vi "Garland_SB parse navigation string.vi"(6 "Header":string="T", 8 "Nav String":string="$,G,43,13,230,P,10,20,120,T,10,10,330,L,14,36,110,A,3,5,B,7,8,C,16,20,D,-1,-1,S,08,12,234\r") -> (0 "Valid?":bool, 1 "angle":i32, 2 "y":i32, 3 "x":i32)   [LabVIEW 2013]
doc: "This VI will parse the Tug navigation string for the Tug letters, A for example, and the time, T. It returns a cluster with the Tug / Time and three values as decimals."
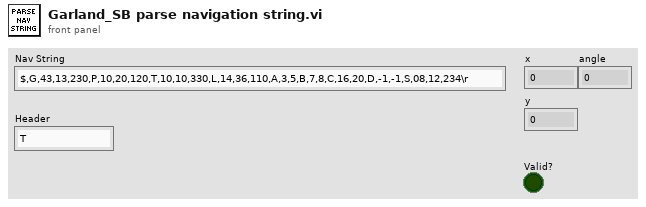
[diagram p1: front panel]
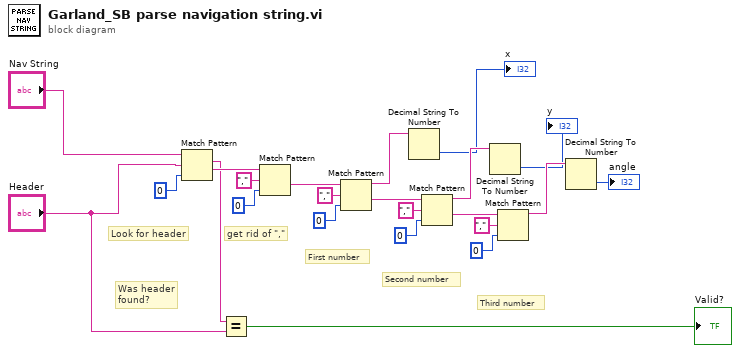
[diagram p0: block diagram]
diagram:
  # "Was header\nfound?"
  # "Third number"
  # "Second number"
  # "First number"
  # "get rid of \",\""
  # "Look for header"
  n1 = Match Pattern(string="Nav String", regular expression="Header", offset (0)=0) -> (match substring=w6:string, after substring=w8:string)  [unwired: 2 out]
  n2 = Equal?(x=w6, y="Header") -> (x = y?=→"Valid?":bool)
  n3 = Match Pattern(string=w8, regular expression=",", offset (0)=0) -> (after substring=w9:string)  [unwired: 3 out]
  n4 = Match Pattern(string=w9, regular expression=",", offset (0)=0) -> (before substring=w20:string, after substring=w16:string)  [unwired: 2 out]
  n5 = Decimal String To Number(string=w20) -> (number=→"x":i32)  [unwired: 2 in, 1 out]
  n6 = Match Pattern(string=w16, regular expression=",", offset (0)=0) -> (before substring=w17:string, after substring=w12:string)  [unwired: 2 out]
  n7 = Decimal String To Number(string=w17) -> (number=→"y":i32)  [unwired: 2 in, 1 out]
  n8 = Match Pattern(string=w12, regular expression=",", offset (0)=0) -> (before substring=w13:string)  [unwired: 3 out]
  n9 = Decimal String To Number(string=w13) -> (number=→"angle":i32)  [unwired: 2 in, 1 out]
